vi "Launch Feature Test View.vi"(8 "error in (no error)":errorcluster, 11 "Example Controller Actor in":refnum<class "Example Controller.lvclass">) -> (0 "error out":errorcluster, 3 "Example Controller Actor out":refnum<class "Example Controller.lvclass">)   [LabVIEW 2023, in "Example MVC Actors.lvlib" / "Example Controller.lvlib" / "Example Controller.lvclass"]
uses:
  Example Controller.lvclass
  Example View/Example View 2/Example View 2.lvclass
  View/View.lvclass/View.ctl
  View/properties/Write Name.vi
  Controller/Controller.lvclass
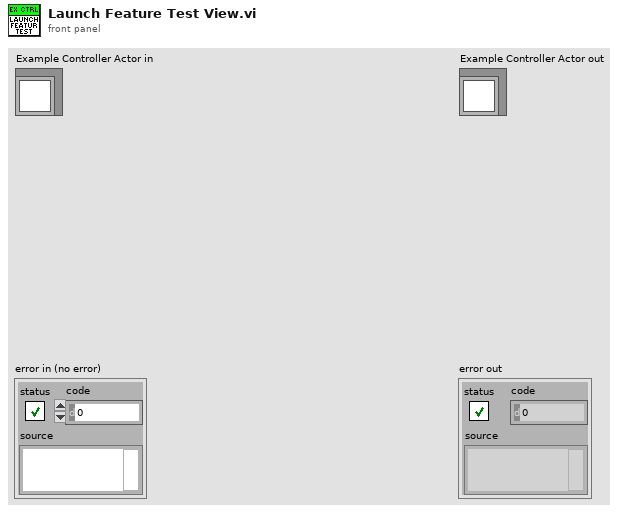
[diagram p1: front panel]
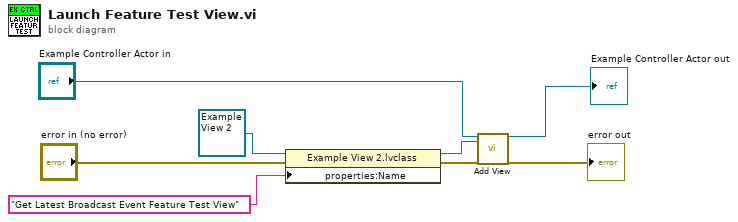
[diagram p0: block diagram]
diagram:
  n1 = property class="Example View 2.lvclass"(reference=refnum<class "Example View 2.lvclass"> refnum ("Example View Actor 2.lvlib:Example View Actor 2.lvclass"), error in="error in (no error)", "properties:Name"="Get Latest Broadcast Event Feature Test View" ("Debug Alias")) -> (reference out=w7:refnum<class "Example View 2.lvclass">, error out=w6:errorcluster)
  n2 = call "Add View.vi"("Controller in"="Example Controller Actor in", "View Actor"=w7, "error in (no error)"=w6) -> ("Controller out"=→"Example Controller Actor out":refnum<class "Example Controller.lvclass">, "error out"=→"error out":errorcluster)  [unwired: 14 in, 1 out]
